vi "RegisterPoll_1298R.vi"(7 "Timeout (ms)":i32=500, 8 "error in (no error)":errorcluster, 9 "Polling Notifier":refnum<notifier>, 11 "Main App Queue":refnum<queue>) -> (0 "error out":errorcluster)   [LabVIEW 2010]
doc: "This VI polls the Lead-off Status Registers of the device.\n\nSee block diagram for details"
uses:
  <userlib>/Common/Queue with Cluster/TYP_Queue Cluster Element.ctl
  Controls/Misc/TYP_PollingStatus.ctl
  Estyx/TYP_ADS1298REstyx File Enum.ctl
  lib_1298/Styx/lvstyx/Read/lvstyx_read_all_path_hex.vi
  <userlib>/Common/Queue with Cluster/Enqueue - ClusterBoth.vi
  lib_1298/lib1299.lvlib
panel:
  out "LOFF_STATN":bool[](array[boolean]) caption="Negative\nElectrode"
  out "LOFF_STATP":bool[](array[boolean]) caption="Positive\nElectrode"
  out "Quit":bool
  out "PolLOFF":bool
  in  "Read Status Registers":bool=TRUE
  # "IN8x"
  # "IN7x"
  # "IN6x"
  # "IN5x"
  # "IN4x"
  # "IN3x"
  # "IN2x"
  # "IN1x"
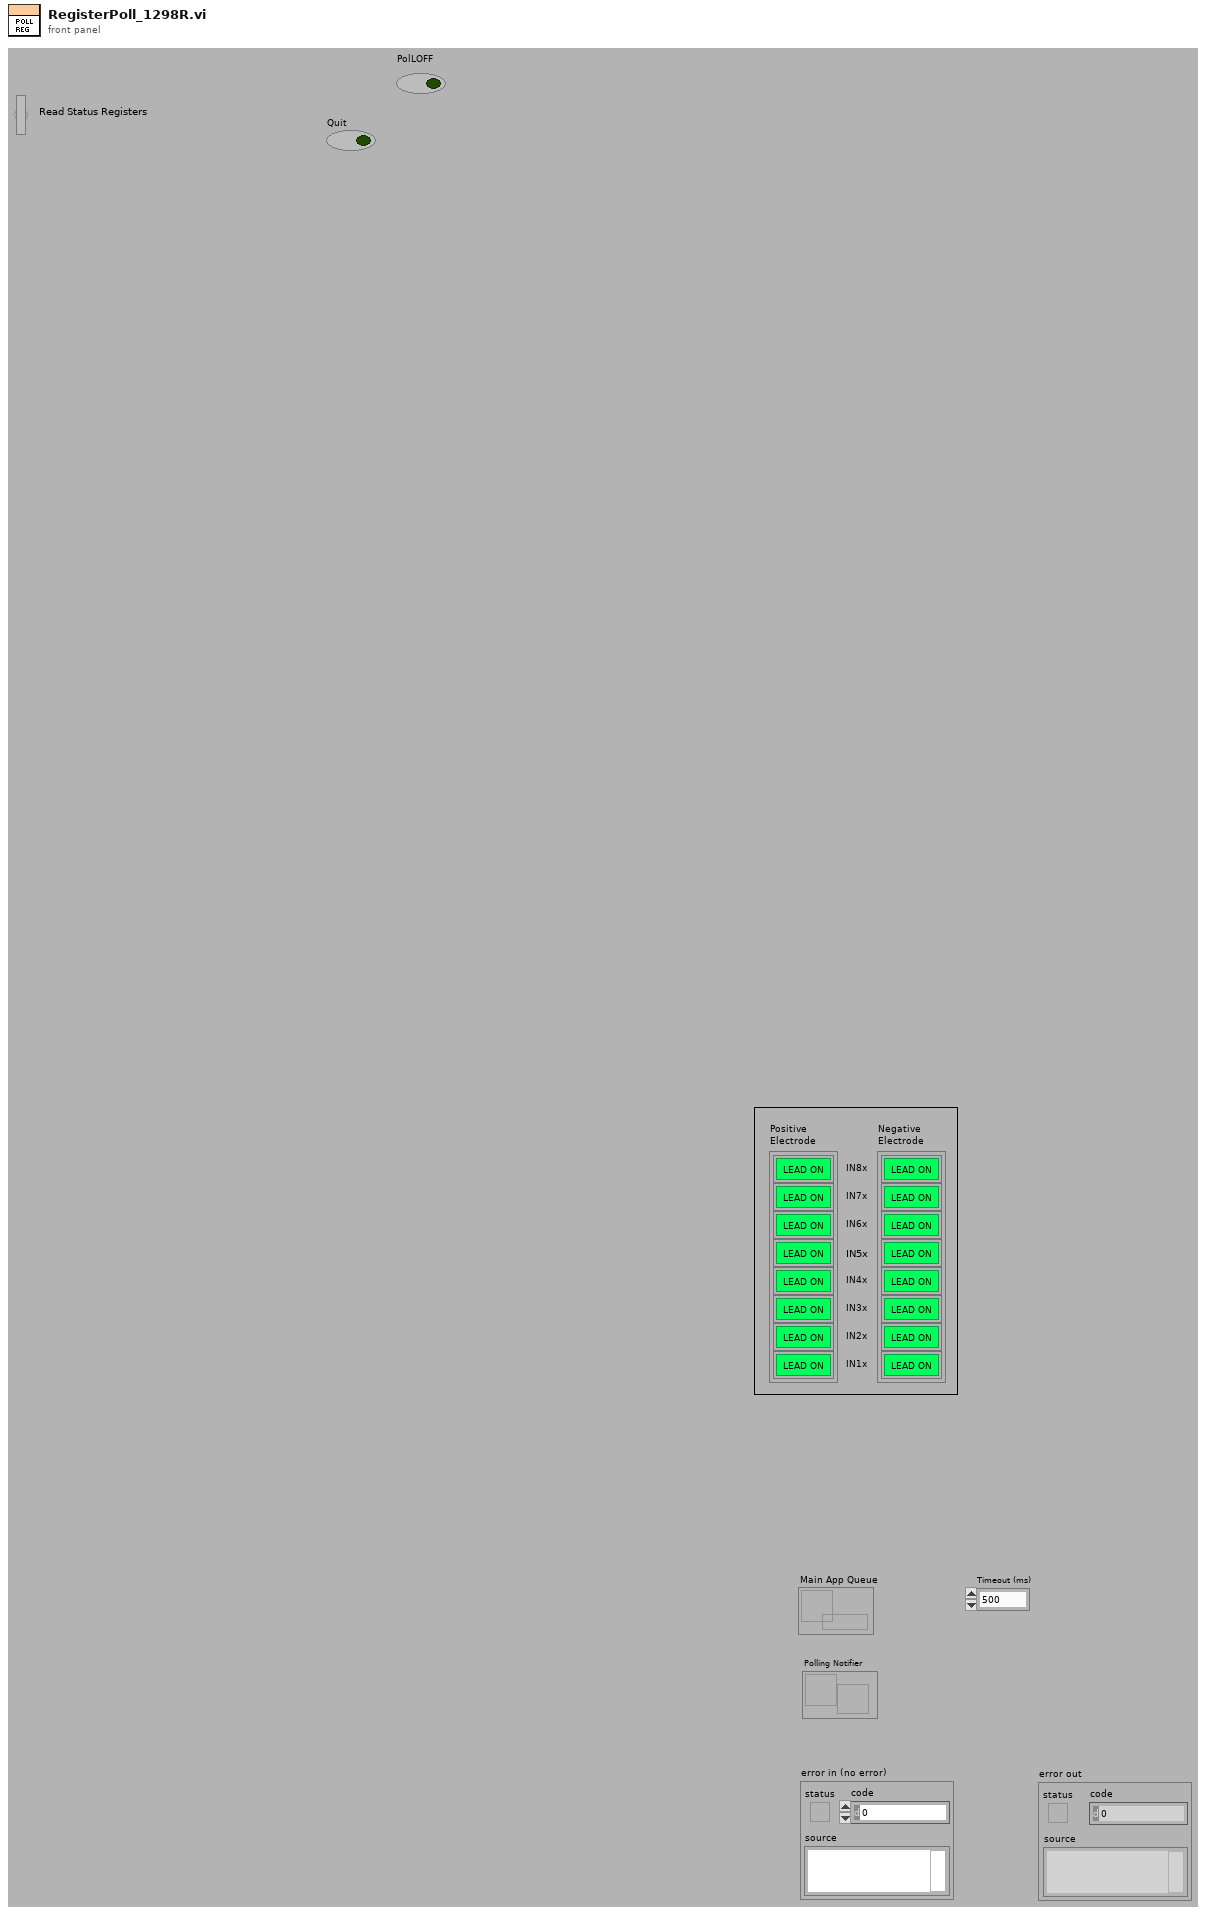
[diagram p1: front panel]
types:
  T1 = typedef "TYP_PollingStatus.ctl" = enum16{"Init", "Start", "Stop", "Pause", "Resume"}
  T2 = typedef "TYP_ADS1298REstyx File Enum.ctl" = enum16{"|version", "|id", "ads1298evm|blocksize_samples", "ads1298evm|acquire", "ads1298evm|data", "ads1298evm|simresp", "conf|ch1set", "conf|ch2set", "conf|ch3set", "conf|ch4set", "conf|ch5set", "conf|ch6set", "conf|ch7set", "conf|ch8set", "conf|config1", "conf|config2", "conf|config3", "conf|devid", "conf|gpio", "conf|loff", "conf|loffflip", "conf|loffsensn", "conf|loffsensp", "conf|loffstatn", "conf|loffstatp", "conf|pace", "conf|resp", "conf|rldsensn", "conf|rldsensp", "conf|reset", "conf|sleep", "conf|config4", "conf|wct1", "conf|wct2", "led|dp", "led|seg", "led|ch", "mmb0|pll", "mmb0|clkout", "mmb0|clkfreq"}
  T3 = enum32{"Invalid", "Standard", "Closed", "Hidden", "Minimized", "Maximized"}
  T4 = enum32{"Invalid", "Default", "Floating", "Floating/Auto-Hide", "Modal"}
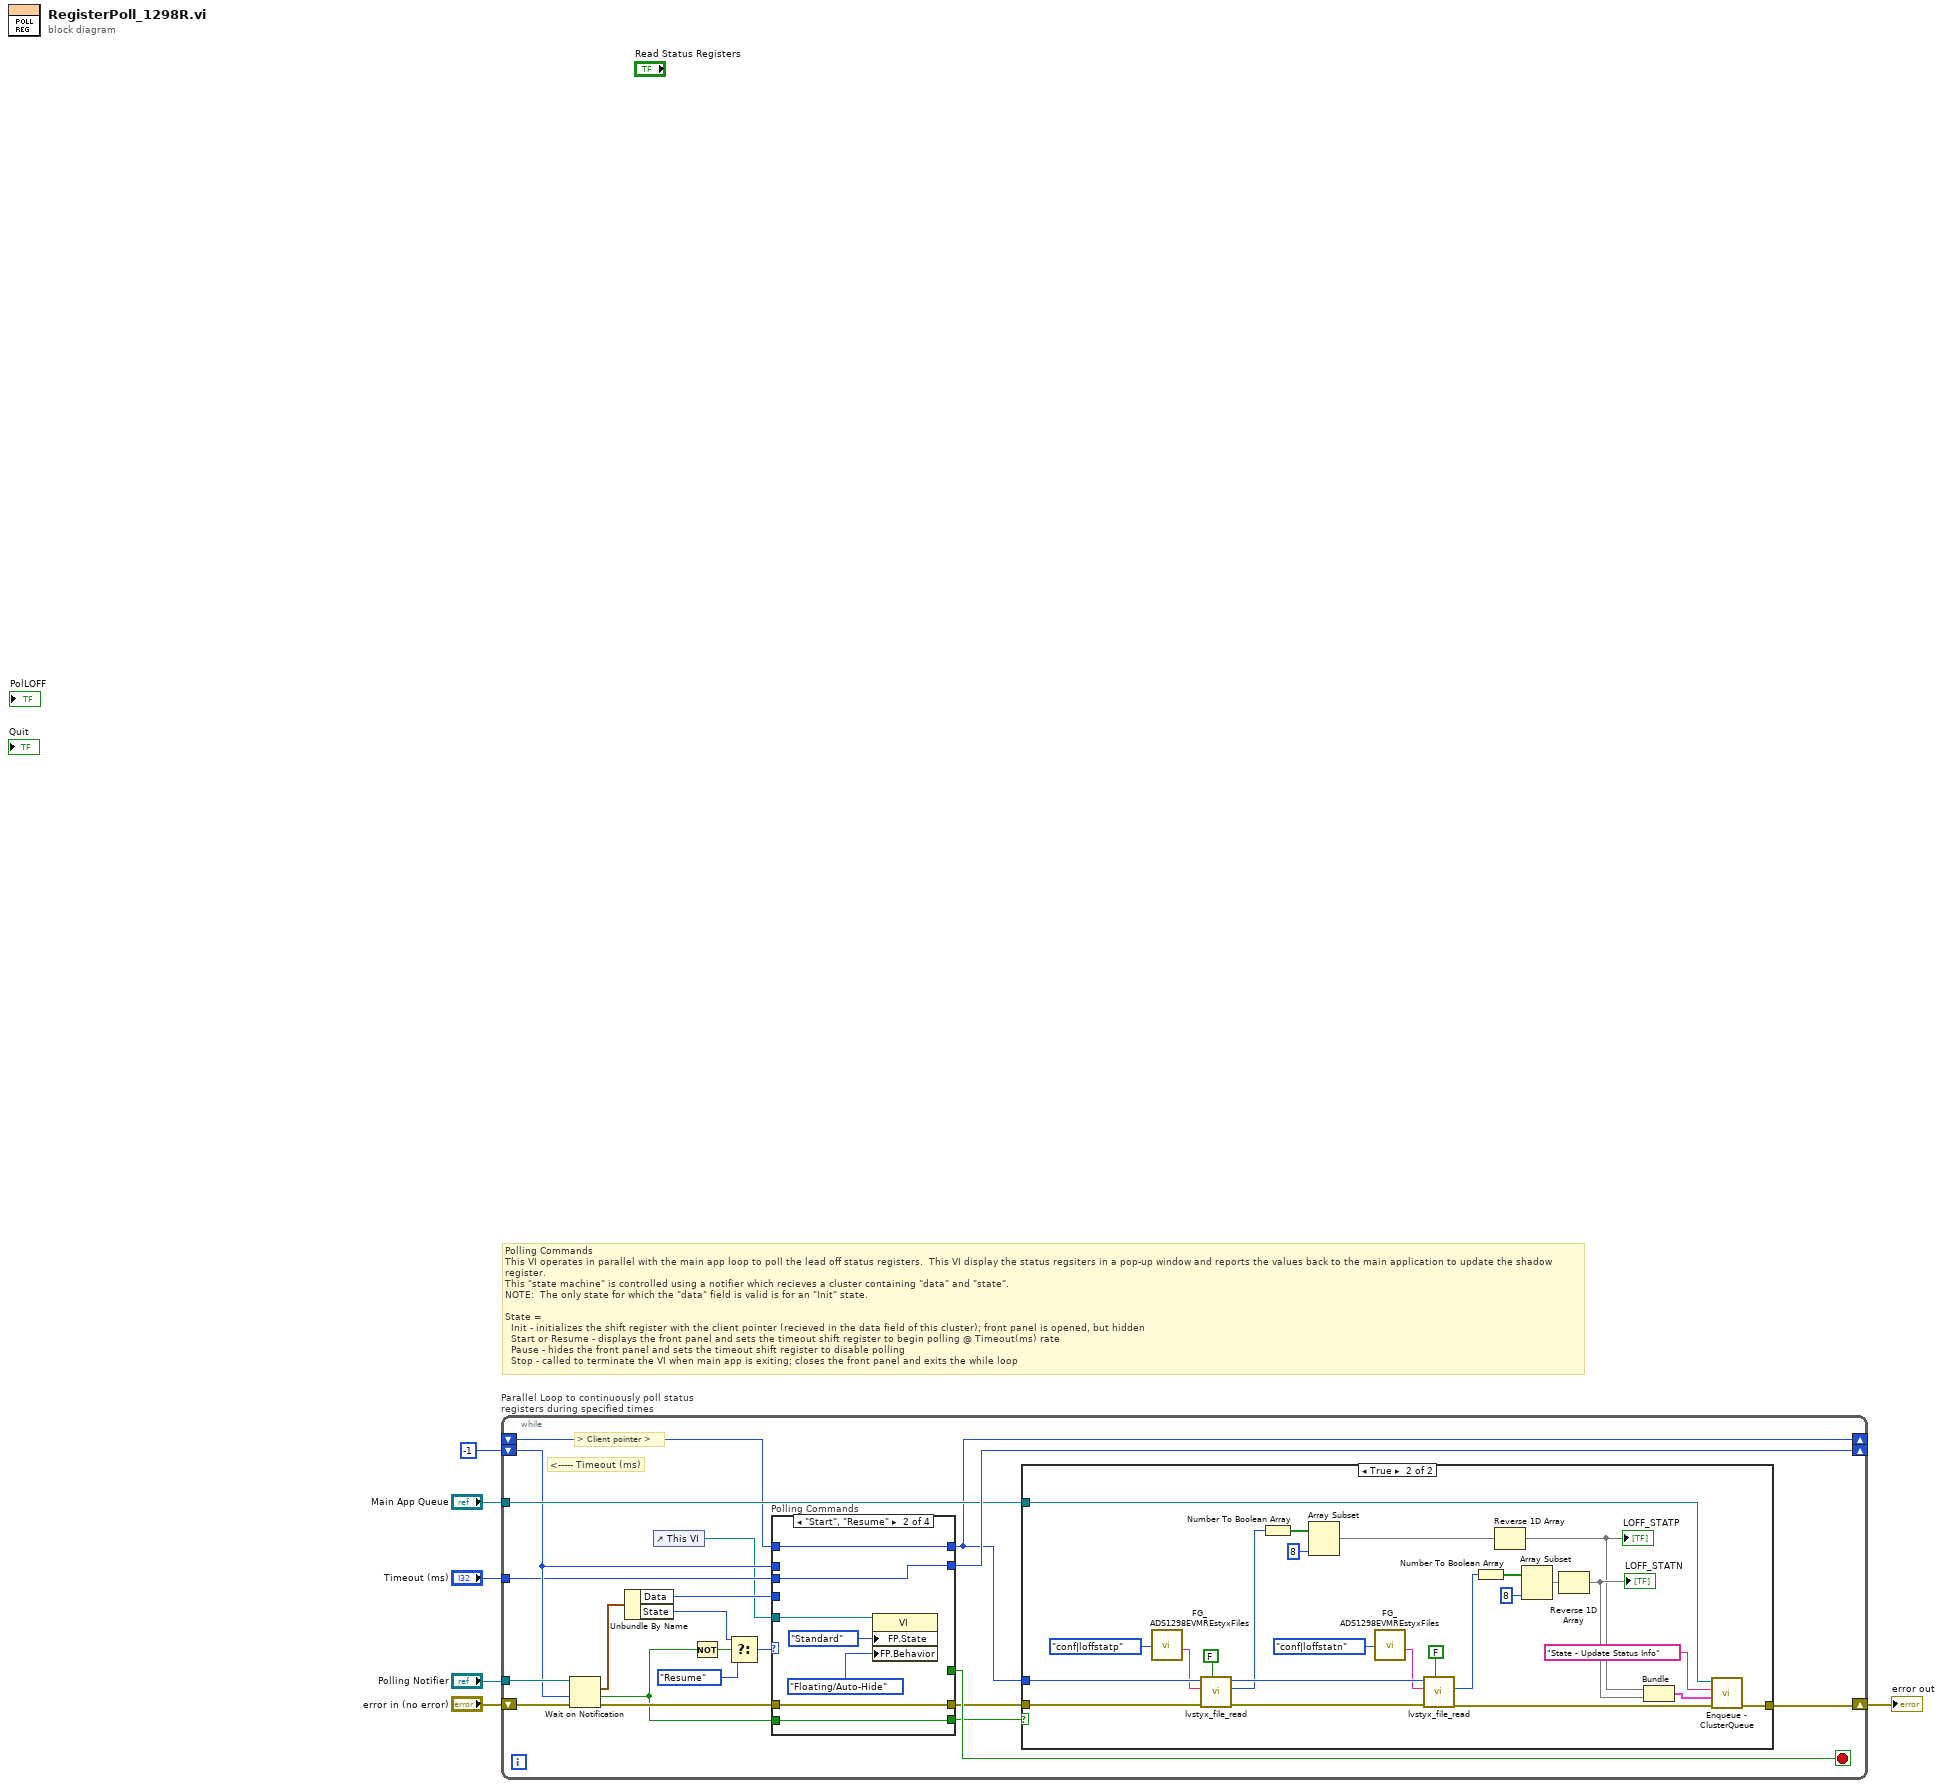
[diagram p0: block diagram]
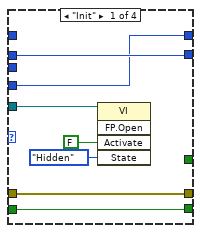
[diagram p3: hidden frame]
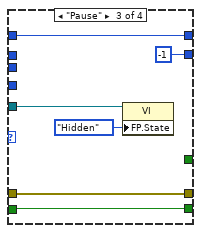
[diagram p4: hidden frame]
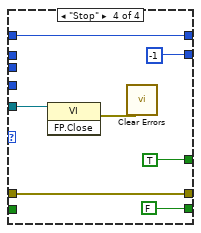
[diagram p5: hidden frame]
diagram:
  # "Polling Commands\nThis VI operates in parallel with the main app loop to poll the lead off status registers.  This VI display the status regsiters in a pop-up window and reports the values back to the main application to update the shadow register.\nThis \"state machine\" is controlled using a notifier which recieves a cluster containing \"data\" and \"state\".\nNOTE:  The only state for which the \"data\" field is valid is for an \"Init\" state.\n\nState =\n  Init - initializes the shift register with the client pointer (recieved in the data field of this cluster); front panel is opened, but hidden\n  Start or Resume - displays the front panel and sets the timeout shift register to begin polling @ Timeout(ms) rate\n  Pause - hides the front panel and sets the timeout shift register to disable polling\n  Stop - called to terminate the VI when main app is exiting; closes the front panel and exits the while loop"
  n1 = while "Parallel Loop to continuously poll status registers during specified times" {
    tunnel: "Main App Queue" -> [w21]
    shift-right: [w7] -> w3
    shift-left: "error in (no error)" -> [w27]
    tunnel: "Polling Notifier" -> [w25]
    shift-right: [w24] -> _
    shift-left: -1 -> [w20]
    shift-right: [w19] -> _
    shift-left: _ -> [w15]
    tunnel: "Timeout (ms)" -> [w16]
    stop <- w23 stop-if-true
    # "<----- Timeout (ms)"
    # "> Client pointer >"
    n2 = Wait on Notification(notifier=w25, timeout in ms (-1)=w20, error in (no error)=w27) -> (notification=w18:cluster{"State":T1, "Data":i32}, timed out?=w9:bool, error out=w26:errorcluster)  [unwired: 2 out]
    n3 = Unbundle By Name(w18) -> ("Data"=w17:i32, "State"=w13:T1)
    n4 = control-ref of="This VI"() -> (w10:refnum<vi>)
    n5 = Not(x=w9) -> (.not. x?=w14:bool)
    n6 = Select(t=w13, s=w14, f=TYP_PollingStatus."Resume") -> (s? t:f=w12:T1)
    n7 = case "Polling Commands" shown="\"Start\", \"Resume\"" w12 {
      tunnel: w26 -> [w59 w67 w72 w79]
      tunnel: [w59 w67 w72 w79] -> w22
      tunnel: w16 -> [_ w66 _ _]
      tunnel: w20 -> [w60 _ _ _]
      tunnel: [w60 w66 -1 ("Timeout (ms)") -1 ("Timeout (ms)")] -> w24
      tunnel: [_ _ _ TRUE] -> w23
      tunnel: [w58 w65 w71 w77] -> w19
      tunnel: w17 -> [w58 _ _ _]
      tunnel: w15 -> [_ w65 w71 w77]
      tunnel: w10 -> [w57 w63 w70 w76]
      tunnel: w9 -> [w54 w61 w68 _]
      tunnel: [w54 w61 w68 FALSE] -> w8
      frame "Init" {
        n8 = invoke class="VI" method="FP.Open"(reference=w57, "Activate"=FALSE ("Activate?"), "State"=T3."Hidden") -> ()  [unwired: 2 in, 5 out]
      }
      frame "Start", "Resume" {
        n9 = property class="VI"(reference=w63, "FP.State"=T3."Standard" ("Front Panel Window:State"), "FP.Behavior"=T4."Floating/Auto-Hide" ("Front Panel Window:Behavior")) -> ()  [unwired: 1 in, 2 out]
      }
      frame "Pause" {
        n10 = property class="VI"(reference=w70, "FP.State"=T3."Hidden" ("Front Panel Window:State")) -> ()  [unwired: 1 in, 2 out]
      }
      frame "Stop" {
        n11 = invoke class="VI" method="FP.Close"(reference=w76) -> (error out=w74:errorcluster)  [unwired: 2 in, 2 out]
        n12 = call <vilib>:"Clear Errors.vi"("error in (no error)"=w74) -> ()  [unwired: 7 out]
      }
    }
    n13 = case shown="True" w8 {
      tunnel: w22 -> [w28 w53]
      tunnel: [w28 w43] -> w7
      tunnel: w21 -> [_ w41]
      tunnel: w19 -> [_ w52]
      frame False {
      }
      frame True {
        n14 = call "FG_ADS1298EVMREstyxFiles.vi"("Storage Info"=TYP_ADS1298REstyx_File_Enum."conf|loffstatp" ("Styx File Tags - Enum")) -> ("File Path"=w29:string)  [unwired: 2 in, 8 out]
        n15 = call-poly "lvstyx_file_read.vi"("Log? (T)"=FALSE ("Notify? (F)"), "error in (no error)"=w53, "path"=w29, "client ptr"=w52) -> ("error out"=w49:errorcluster, "uint32"=w30:u32, "dup client ptr"=w48:u32)  [unwired: 5 in]
        n16 = Number To Boolean Array(number=w30) -> (Boolean array=w47:bool[])
        n17 = Array Subset(array=w47, length=8) -> (w39:bool[])  [unwired: 1 in]
        n18 = call "FG_ADS1298EVMREstyxFiles.vi"("Storage Info"=TYP_ADS1298REstyx_File_Enum."conf|loffstatn" ("Styx File Tags - Enum")) -> ("File Path"=w32:string)  [unwired: 2 in, 8 out]
        n19 = call-poly "lvstyx_file_read.vi"("Log? (T)"=FALSE ("Notify? (F)"), "error in (no error)"=w49, "path"=w32, "client ptr"=w48) -> ("error out"=w42:errorcluster, "uint32"=w31:u32)  [unwired: 5 in, 1 out]
        n20 = Number To Boolean Array(number=w31) -> (Boolean array=w44:bool[])
        n21 = Reverse 1D Array(array=w39) -> (reversed array=w33:bool[])
        "LOFF_STATP" <- w33
        n22 = Array Subset(array=w44, length=8) -> (w38:bool[])  [unwired: 1 in]
        n23 = Reverse 1D Array(array=w38) -> (reversed array=w34:bool[])
        "LOFF_STATN" <- w34
        n24 = Bundle(w33, w34) -> (w37:cluster{bool[], bool[]})  [unwired: 1 out]
        n25 = call-poly <userlib>:"Enqueue - ClusterQueue.vi"("error in (no error)"=w42, "Data"=w37, "Command"="State - Update Status Info", "Queue with Cluster Reference"=w41) -> ("error out"=w43:errorcluster)  [unwired: 2 in, 5 out]
      }
    }
  }
  "error out" <- w3
